vi "XY Graph Get Scale Labels.vi"(8 "Error In":errorcluster, 11 "XYGraph in":T1) -> (0 "Error Out":errorcluster, 1 "Y Scale Labels":string[](array[string]), 2 "X Scale Labels":string[](array[string]), 3 "XYGraph out":T1, 4 "# Y Scales":i32, 6 "# X Scales":i32)   [LabVIEW 2021, in "XY Graph Add-Ons.lvlib"]
uses:
  XY Graph Add-Ons.lvlib
  XY Graph Refnum.ctl
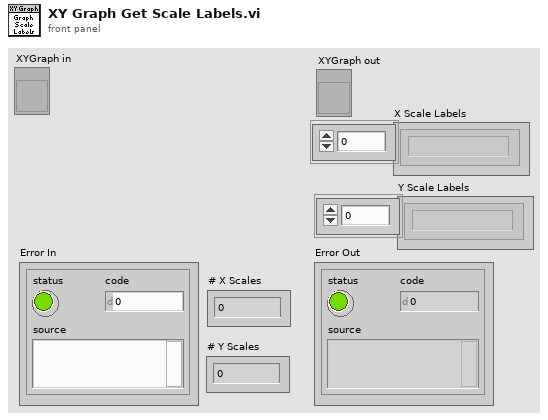
[diagram p1: front panel]
types:
  T1 = typedef "XY Graph Add-Ons.lvlib/XY Graph Refnum.ctl" = refnum<vi>
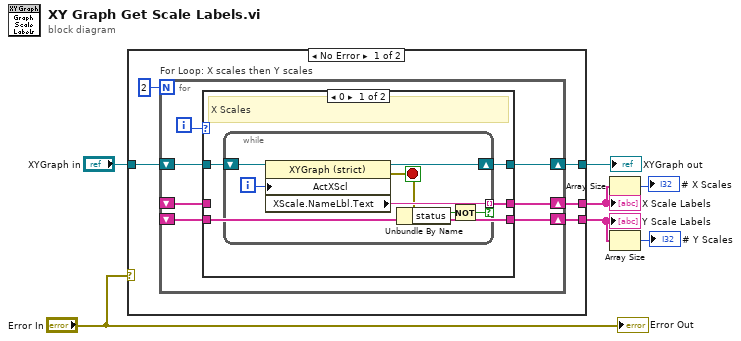
[diagram p0: block diagram]
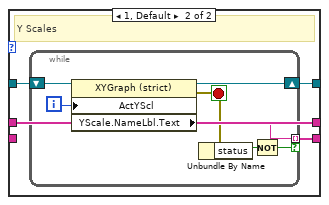
[diagram p2: hidden frame]
diagram:
  n1 = case shown="No Error" "Error In" {
    tunnel: "XYGraph in" -> [w12 w42]
    tunnel: [w11 w42] -> w6
    tunnel: [w9 _] -> w4
    tunnel: [w8 _] -> w2
    frame No Error {
      n2 = for "For Loop: X scales then Y scales" {
        N: 2 -> [_]
        shift-right: [w18] -> w11
        shift-left: w12 -> [w19]
        shift-right: [w16] -> w9
        shift-left: _ -> [w15]
        shift-right: [w14] -> w8
        shift-left: _ -> [w13]
        i -> [w17]
        n3 = case shown="0" w17 {
          tunnel: w19 -> [w23 w34]
          tunnel: [w22 w33] -> w18
          tunnel: [w21 w32] -> w16
          tunnel: w15 -> [_ w32]
          tunnel: [w20 w31] -> w14
          tunnel: w13 -> [w20 _]
          frame 0 {
            # "X Scales"
            n4 = while {
              shift-right: [w29] -> w22
              shift-left: w23 -> [w30]
              tunnel: [w27] -> w21 mode=indexing if=w24
              i -> [w28]
              stop <- w26 stop-if-true
              n5 = property class="XYGraph (strict)"(reference=w30, "ActXScl"=w28) -> (reference out=w29:T1, error out=w26:errorcluster, "XScale.NameLbl.Text"=w27:string)  [unwired: 1 in]
              n6 = Unbundle By Name(w26) -> ("status"=w25:bool)
              n7 = Not(x=w25) -> (.not. x?=w24:bool)
            }
          }
          frame 1, Default {
            # "Y Scales"
            n8 = while {
              shift-right: [w40] -> w33
              shift-left: w34 -> [w41]
              tunnel: [w36] -> w31 mode=indexing if=w35
              i -> [w39]
              stop <- w38 stop-if-true
              n9 = property class="XYGraph (strict)"(reference=w41, "ActYScl"=w39) -> (reference out=w40:T1, error out=w38:errorcluster, "YScale.NameLbl.Text"=w36:string)  [unwired: 1 in]
              n10 = Unbundle By Name(w38) -> ("status"=w37:bool)
              n11 = Not(x=w37) -> (.not. x?=w35:bool)
            }
          }
        }
      }
    }
    frame Error {
    }
  }
  "XYGraph out" <- w6
  "X Scale Labels" <- w4
  "Y Scale Labels" <- w2
  n12 = Array Size(array=w4) -> (size(s)=→"# X Scales":i32)
  n13 = Array Size(array=w2) -> (size(s)=→"# Y Scales":i32)
  "Error Out" <- "Error In"
